vi "NPC3SG Move Axis To.vi"(0 "Drive Visa Name":refnum<visa-resource-name>="COM5", 1 "Running":refnum<vi>, 2 "Axis":i32=1 min=0 max=2 step=1, 3 "Drive Set":dbl=10.0 caption="Target (µm)" min=10.0 max=160.0 step=0.1 format="%.3f") -> (7 "Send Error":errorcluster caption="Fehler (Ausgang)")   [LabVIEW 2010]
uses:
  drivers/Newport NPC3SG/SubNPC3SG.llb/device variables.vi
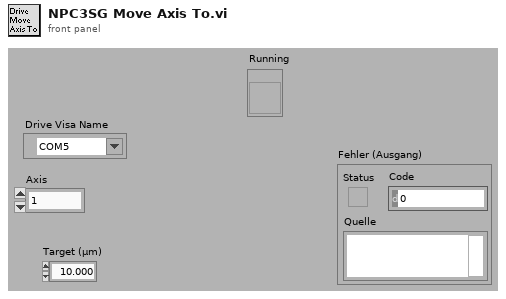
[diagram p1: front panel]
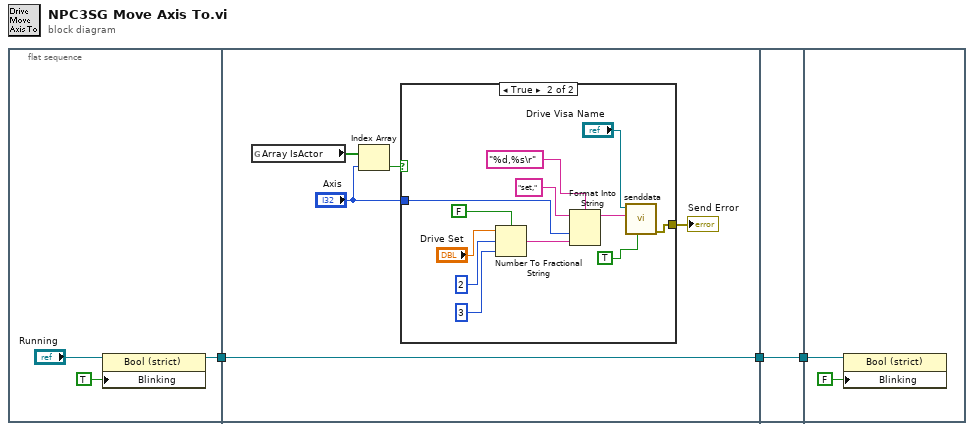
[diagram p0: block diagram]
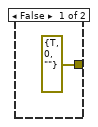
[diagram p2: hidden frame]
diagram:
  n1 = flat-sequence {
    tunnel: [w4] -> w3
    tunnel: [w11] -> w2
    tunnel: w3 -> [w11]
    tunnel: w2 -> [w25]
    tunnel: [w25] -> w1
    tunnel: w1 -> [w27]
    frame #0 {
      n2 = property class="Bool (strict)"(reference="Running", "Blinking"=TRUE ("Blinkend")) -> (reference out=w4:refnum<vi>)  [unwired: 1 in, 1 out]
    }
    frame #1 {
      n3 = global read "device variables.vi" "Array IsActor"() -> (w10:bool[])
      n4 = Index Array(array=w10, index="Axis") -> (element=w9:bool)
      n5 = case shown="True" w9 {
        tunnel: "Axis" -> [_ w16]
        tunnel: [errorcluster {"status"=TRUE, "code"=0, "source"=""} ("error out") w15] -> w8
        frame False {
        }
        frame True {
          n6 = Number To Fractional String(use system decimal point (T)=FALSE ("Systemdezimalzeichen verwenden (T)"), number="Drive Set", width (-)=i16 2 ("Breite (-)"), precision (6)=i16 3 ("Genauigkeit (6)")) -> (F-format string=w22:string)
          n7 = Format Into String(format string="%d,%s\r", initial string="set,", w16, w22) -> (resulting string=w23:string)  [unwired: 1 in, 1 out]
          n8 = call "senddata.vi"("read ERR"=TRUE, "writebuffer"=w23, "VISA-Ressourcen-Name"="Drive Visa Name") -> ("error out"=w15:errorcluster)  [unwired: 6 in, 2 out]
        }
      }
      "Send Error" <- w8
    }
    frame #2 {
    }
    frame #3 {
      n9 = property class="Bool (strict)"(reference=w27, "Blinking"=FALSE ("Blinkend")) -> ()  [unwired: 1 in, 2 out]
    }
  }
